vi "Bytes to MB.vi"(3 "Metrics: Data Size":u32) -> (1 "MB":dbl)   [LabVIEW 2023, in "VIDoc Parsing.lvlib"]
uses:
  VIDoc Parsing.lvlib
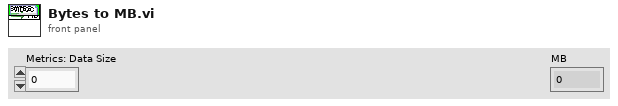
[diagram p1: front panel]
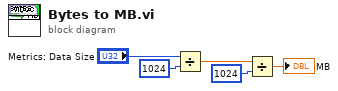
[diagram p0: block diagram]
diagram:
  n1 = Divide(x="Metrics: Data Size", y=u32 1024) -> (x/y=w3:dbl)
  n2 = Divide(x=w3, y=u32 1024) -> (x/y=→"MB":dbl)
